vi "Bras.vi"(0 "Commande":bool) -> ()   [LabVIEW 2018]
uses:
  <vilib>/Rock Robotics/WPI/ThirdParty/Phoenix-LabVIEW/Motor Controller/Controls/CTRE_Phoenix_MotorControl_ControlMode.ctl
  <vilib>/Rock Robotics/WPI/DriverStation/WPI_DriverStationRobotMode2.ctl
  <vilib>/Rock Robotics/WPI/ThirdParty/Phoenix-LabVIEW/Motor Controller/Get/CTRE_Phoenix_MotorController_GetSelectedSensorData.vi
  <vilib>/Rock Robotics/Network Tables/NT Write Number.vi
  <vilib>/Rock Robotics/Network Tables/NT Read Boolean.vi
  Robot Global Data.vi
  <vilib>/Rock Robotics/Network Tables/NT Write Boolean.vi
  <vilib>/Rock Robotics/WPI/Utilities/WPI_GetSetVariantRefNum.vi
panel:
  in  "vitesse descendre":dbl=-0.215618
  in  "vitesse monte":dbl=0.4
  in  "pos. bas.":dbl=-255.0
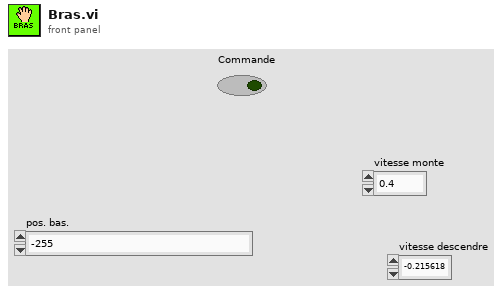
[diagram p1: front panel]
types:
  T1 = typedef "CTRE_Phoenix_MotorControl_ControlMode.ctl" = u16
  T2 = typedef "WPI_MotorControlDeviceRef.ctl" = cluster{"DeviceStatus":errorcluster, "Type":T3, "PWM":cluster{"PWM Channel":T4, "DeadBand":T5}, "CAN":cluster{"Device Number":u8, "SetOutput VI Ref":variant, "GetOutput VI Ref":variant, "Enable VI Ref":variant, "Disable VI Ref":variant, "Data":variant}, "Invert":bool, "DIO PWM":cluster{"PWM \"Enable\" Channel":T4, "DIOChannel":T6, "PWM Rate":dbl}}
  T3 = typedef "WPI_MotorControlType.ctl" = enum16{"PWM", "CAN", "DIO PWM"}
  T4 = typedef "FPGA_DIOPWMChannel.ctl" = enum8{"PWM 0", "PWM 1", "PWM 2", "PWM 3", "PWM 4", "PWM 5", "PWM 6", "PWM 7", "PWM 8", "PWM 9", "PWM MXP 0", "PWM MXP 1", "PWM MXP 2", "PWM MXP 3", "PWM MXP 4", "PWM MXP 5", "PWM MXP 6", "PWM MXP 7", "PWM MXP 8", "PWM MXP 9", "Invalid"}
  T5 = typedef "WPI_PWMDeadband.ctl" = cluster{"Name":string, "maxPositivePwm":i32, "minPositivePwm":i32, "centerPwm":i32, "maxNegativePwm":i32, "minNegativePwm":i32, "angularRange":u16}
  T6 = typedef "FPGA_DIOChannel.ctl" = enum8{"DIO 0", "DIO 1", "DIO 2", "DIO 3", "DIO 4", "DIO 5", "DIO 6", "DIO 7", "DIO 8", "DIO 9", "DIO MXP 0", "DIO MXP 1", "DIO MXP 2", "DIO MXP 3", "DIO MXP 4", "DIO MXP 5", "DIO MXP 6", "DIO MXP 7", "DIO MXP 8", "DIO MXP 9", "DIO MXP 10", "DIO MXP 11", "DIO MXP 12", "DIO MXP 13", "DIO MXP 14", "DIO MXP 15", "SPI Port CS1", "SPI Port CS2", "SPI Port CS3", "SPI Port MISO", "SPI Port MOSI", "Invalid"}
  T7 = typedef "WPI_DriverStationRobotMode2.ctl" = enum16{"Autonomous Disabled", "Autonomous Enabled", "Teleop Disabled", "Teleop Enabled", "Disconnected", "Finish", "Test Disabled", "Test Enabled", "Emergency Stopped"}
  T8 = typedef "WPI_SwitchDevRef.ctl" = cluster{"DevStatus":errorcluster, "DIO Channel":T6, "CntIndex":T9, "Normally Closed":bool}
  T9 = typedef "FPGA_CounterCtrSystemIndex.ctl" = enum8{"Ctr 0", "Ctr 1", "Ctr 2", "Ctr 3", "Ctr 4", "Ctr 5", "Ctr 6", "Ctr 7", "Invalid"}
  T10 = typedef "WPI_JoystickDevRef.ctl" = cluster{"Device":T11}
  T11 = typedef "WPI_JoystickDeviceEnum.ctl" = enum16{"USB 0", "USB 1", "USB 2", "USB 3", "USB 4", "USB 5"}
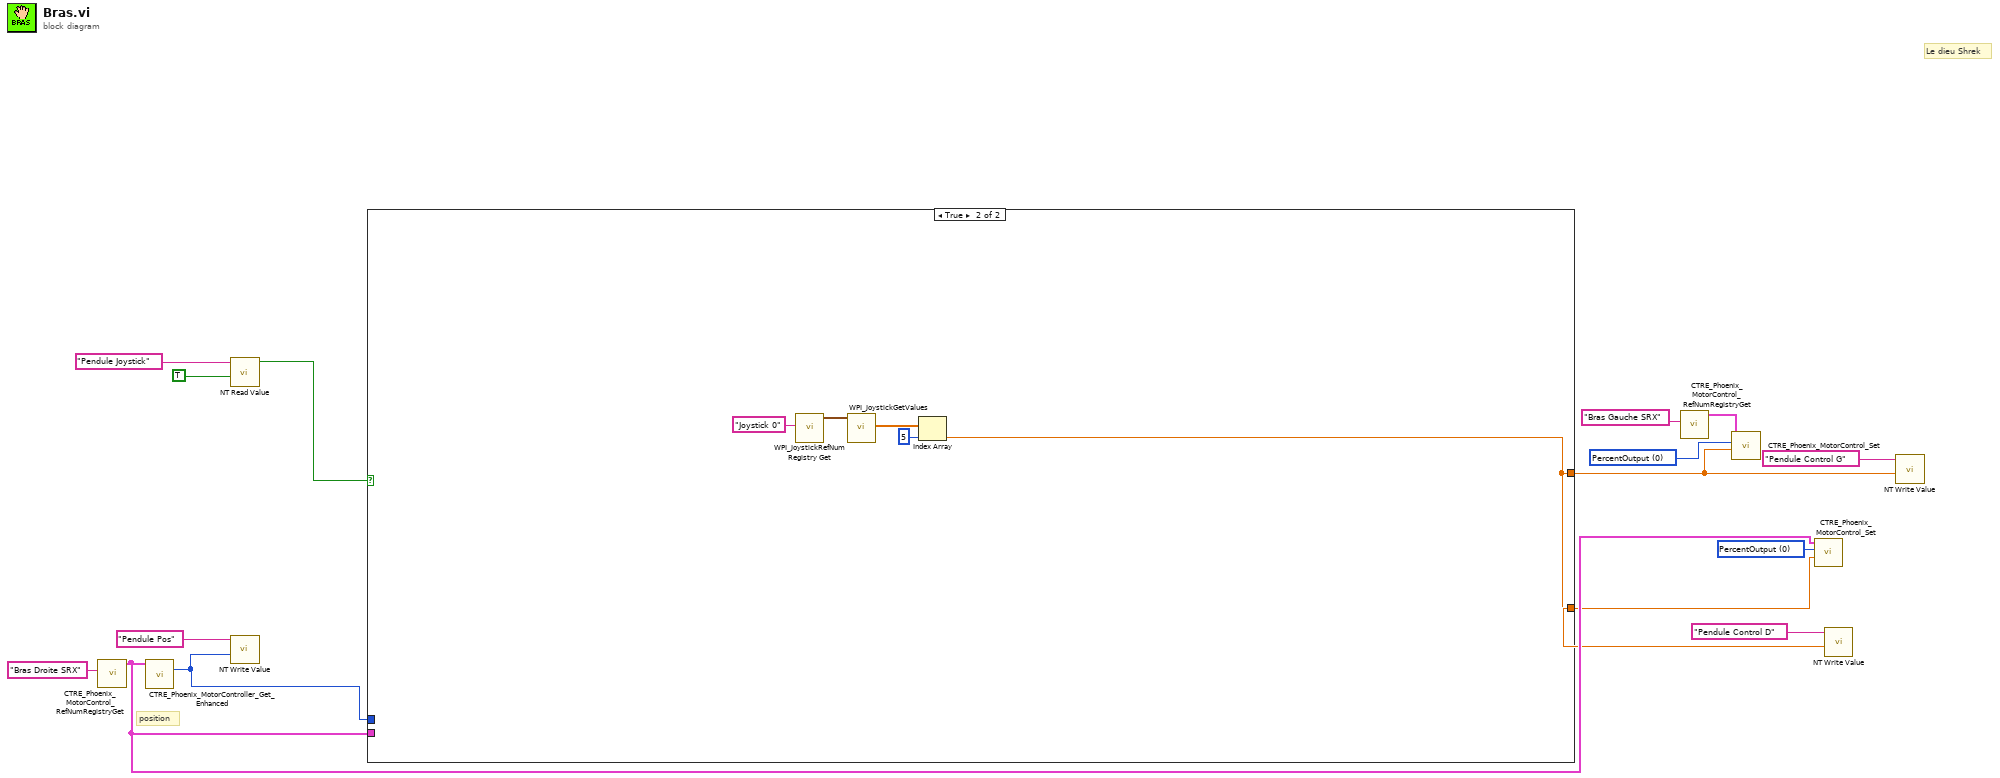
[diagram p0: block diagram]
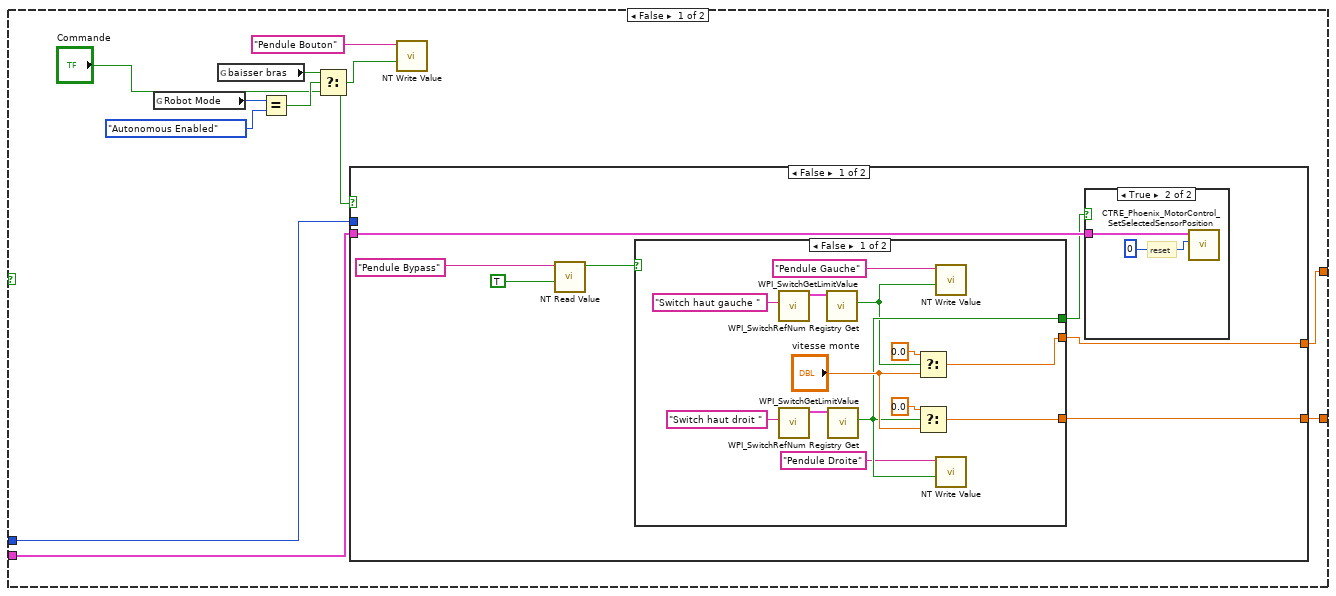
[diagram p2: hidden frame]
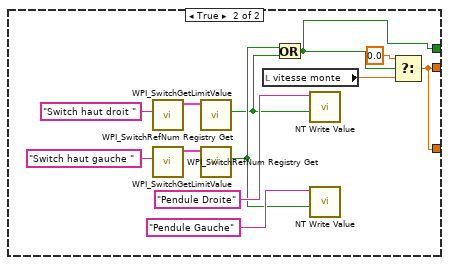
[diagram p3: hidden frame]
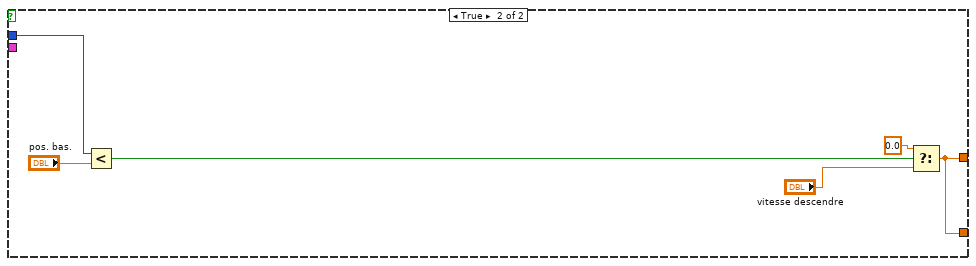
[diagram p5: hidden frame]
diagram:
  w8 = T1 0 items=["PercentOutput"=0, "Position"=1, "Velocity"=2, "Current"=3, "Follower"=5, "MotionProfile"=6, "MotionMagic"=7, "MotionProfileArc"=10, "Disabled"=15] ("Control Mode")
  w11 = T1 0 items=["PercentOutput"=0, "Position"=1, "Velocity"=2, "Current"=3, "Follower"=5, "MotionProfile"=6, "MotionMagic"=7, "MotionProfileArc"=10, "Disabled"=15] ("Control Mode")
  # "position"
  # "Le dieu Shrek"
  n1 = call <vilib>:"CTRE_Phoenix_MotorControl_RefNumRegistryGet.vi"("refnum name"="Bras Droite SRX") -> ("PhoenixMotorControlDevRef"=w14:T2)  [unwired: 9 in, 1 out]
  n2 = call-poly <vilib>:"CTRE_Phoenix_MotorController_Get_Enhanced.vi"("PhoenixMotorControlDevRef"=w14) -> ("Position (Raw Sensor Units)"=w13:i32)  [unwired: 11 in, 3 out]
  n3 = call-poly <vilib>:"NT Read Value.vi"("Default Value"=TRUE, "Name"="Pendule Joystick") -> ("Boolean"=w1:bool)  [unwired: 8 in, 1 out]
  n4 = call-poly <vilib>:"NT Write Value.vi"("Numeric"=w13, "Name"="Pendule Pos") -> ()  [unwired: 9 in, 1 out]
  n5 = case shown="True" w1 {
    tunnel: w14 -> [w26 _]
    tunnel: w13 -> [w20 _]
    tunnel: [w17 w67] -> w5
    tunnel: [w16 w67] -> w4
    frame False {
      n6 = global read "Robot Global Data.vi" "Robot Mode"() -> (w25:T7)
      n7 = global read "Robot Global Data.vi" "baisser bras"() -> (w22:bool)
      n8 = Equal?(x=w25, y=WPI_DriverStationRobotMode2."Autonomous Enabled") -> (x = y?=w23:bool)
      n9 = Select(t=w22, s=w23, f="Commande") -> (s? t:f=w19:bool)
      n10 = case shown="False" w19 {
        tunnel: [w33 w65] -> w17
        tunnel: [w32 w65] -> w16
        tunnel: w20 -> [_ w63]
        tunnel: w26 -> [w31 _]
        frame False {
          n11 = call-poly <vilib>:"NT Read Value.vi"("Default Value"=TRUE, "Name"="Pendule Bypass") -> ("Boolean"=w29:bool)  [unwired: 8 in, 1 out]
          n12 = case shown="False" w29 {
            tunnel: [w41 w48] -> w33
            tunnel: [w40 w48] -> w32
            tunnel: [w37 w47] -> w30
            frame False {
              n13 = call <vilib>:"WPI_SwitchRefNum Registry Get.vi"("refnum name"="Switch haut gauche ") -> ("SwitchDevRef"=w46:T8)  [unwired: 9 in, 1 out]
              n14 = call <vilib>:"WPI_SwitchRefNum Registry Get.vi"("refnum name"="Switch haut droit ") -> ("SwitchDevRef"=w44:T8)  [unwired: 9 in, 1 out]
              n15 = call <vilib>:"WPI_SwitchGetLimitValue.vi"("SwitchDevRef"=w46) -> ("Switch Pressed"=w36:bool)  [unwired: 8 in, 2 out]
              n16 = call <vilib>:"WPI_SwitchGetLimitValue.vi"("SwitchDevRef"=w44) -> ("Switch Pressed"=w37:bool)  [unwired: 8 in, 2 out]
              n17 = Select(t=0.0, s=w36, f="vitesse monte") -> (s? t:f=w41:dbl)
              n18 = Select(t=0.0, s=w37, f="vitesse monte") -> (s? t:f=w40:dbl)
              n19 = call-poly <vilib>:"NT Write Value.vi"("Boolean"=w36, "Name"="Pendule Gauche") -> ()  [unwired: 9 in, 1 out]
              n20 = call-poly <vilib>:"NT Write Value.vi"("Boolean"=w37, "Name"="Pendule Droite") -> ()  [unwired: 9 in, 1 out]
            }
            frame True {
              n21 = call <vilib>:"WPI_SwitchRefNum Registry Get.vi"("refnum name"="Switch haut droit ") -> ("SwitchDevRef"=w55:T8)  [unwired: 9 in, 1 out]
              n22 = call <vilib>:"WPI_SwitchRefNum Registry Get.vi"("refnum name"="Switch haut gauche ") -> ("SwitchDevRef"=w58:T8)  [unwired: 9 in, 1 out]
              n23 = call <vilib>:"WPI_SwitchGetLimitValue.vi"("SwitchDevRef"=w55) -> ("Switch Pressed"=w51:bool)  [unwired: 8 in, 2 out]
              n24 = call <vilib>:"WPI_SwitchGetLimitValue.vi"("SwitchDevRef"=w58) -> ("Switch Pressed"=w52:bool)  [unwired: 8 in, 2 out]
              n25 = local read "vitesse monte"() -> (w49:dbl)
              n26 = Or(x=w52, y=w51) -> (x .or. y?=w47:bool)
              n27 = call-poly <vilib>:"NT Write Value.vi"("Boolean"=w51, "Name"="Pendule Droite") -> ()  [unwired: 9 in, 1 out]
              n28 = call-poly <vilib>:"NT Write Value.vi"("Boolean"=w52, "Name"="Pendule Gauche") -> ()  [unwired: 9 in, 1 out]
              n29 = Select(t=0.0, s=w47, f=w49) -> (s? t:f=w48:dbl)
            }
          }
          n30 = case shown="True" w30 {
            tunnel: w31 -> [_ w59]
            frame False {
            }
            frame True {
              # "reset"
              n31 = call <vilib>:"CTRE_Phoenix_MotorControl_SetSelectedSensorPosition.vi"("New Sensor Position"=0, "PhoenixMotorControlDevRef"=w59) -> ()  [unwired: 8 in, 2 out]
            }
          }
        }
        frame True {
          n32 = Less?(x=w63, y="pos. bas.") -> (x < y?=w62:bool)
          n33 = Select(t=0.0, s=w62, f="vitesse descendre") -> (s? t:f=w65:dbl)
        }
      }
      n34 = call-poly <vilib>:"NT Write Value.vi"("Boolean"=w19, "Name"="Pendule Bouton") -> ()  [unwired: 9 in, 1 out]
    }
    frame True {
      n35 = call <vilib>:"WPI_JoystickRefNum Registry Get.vi"("refnum name"="Joystick 0") -> ("JoystickDevRef"=w70:T10)  [unwired: 1 in, 9 out]
      n36 = call <vilib>:"WPI_JoystickGetValues.vi"("JoystickDevRef"=w70) -> ("Axes"=w69:dbl[])  [unwired: 6 in, 4 out]
      n37 = Index Array(array=w69, index=5) -> (element=w67:dbl)
    }
  }
  n38 = call <vilib>:"CTRE_Phoenix_MotorControl_RefNumRegistryGet.vi"("refnum name"="Bras Gauche SRX") -> ("PhoenixMotorControlDevRef"=w10:T2)  [unwired: 9 in, 1 out]
  n39 = call <vilib>:"CTRE_Phoenix_MotorControl_Set.vi"("Output"=w5, "Control Mode"=w11, "PhoenixMotorControlDevRef"=w10) -> ()  [unwired: 7 in, 2 out]
  n40 = call <vilib>:"CTRE_Phoenix_MotorControl_Set.vi"("Output"=w4, "Control Mode"=w8, "PhoenixMotorControlDevRef"=w14) -> ()  [unwired: 7 in, 2 out]
  n41 = call-poly <vilib>:"NT Write Value.vi"("Numeric"=w4, "Name"="Pendule Control D") -> ()  [unwired: 9 in, 1 out]
  n42 = call-poly <vilib>:"NT Write Value.vi"("Numeric"=w5, "Name"="Pendule Control G") -> ()  [unwired: 9 in, 1 out]
